vi "ShowBinary.vi"(1 "Numeric":u8) -> (0 "resulting string":string)   [LabVIEW 2012]
panel:
  in  "stop":bool
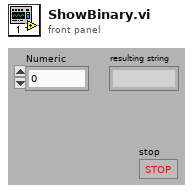
[diagram p1: front panel]
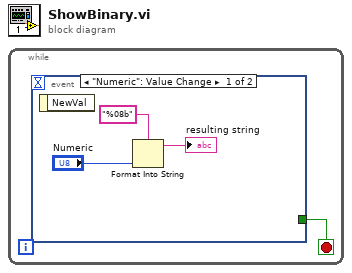
[diagram p0: block diagram]
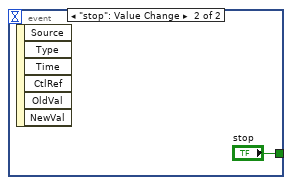
[diagram p2: hidden frame]
diagram:
  n1 = while {
    stop <- w1 stop-if-true
    n2 = event shown="[0] \"Numeric\": Value Change" {
      selector: _ -> [_ _]
      dyn-events: _ -> [_ _]
      timeout: _ -> [_ _]
      tunnel: [_ "stop"] -> w1
      event "Numeric": Value Change {
        n3 = event-data() -> ()  [unwired: 1 in, 1 out]
        n4 = Format Into String(format string="%08b", "Numeric") -> (resulting string=→"resulting string":string)  [unwired: 2 in, 1 out]
      }
      event "stop": Value Change {
        n5 = event-data() -> ()  [unwired: 1 in, 6 out]
      }
    }
  }
